vi "Analyse File to Prep DB.vi"(6 "Dummy Data 2":string, 7 "Dummy fill?":bool, 8 "error in (no error)":errorcluster, 9 "Dummy Data":string, 10 "Delimiter":string, 11 "Txt  file":path) -> (0 "error out":errorcluster, 1 "Value to be inserted":string, 2 "Table Elements":string, 3 "Table Schema":string)   [LabVIEW 2018]
panel:
  out "output array 2":string[][](array[string])
  in  "Quit":bool
  in  "User input Delimiter":string
  in  "Delimiter":enum16{"Tab", "Comma", "Space", "Ohters"}(ring)
  in  "Show":bool
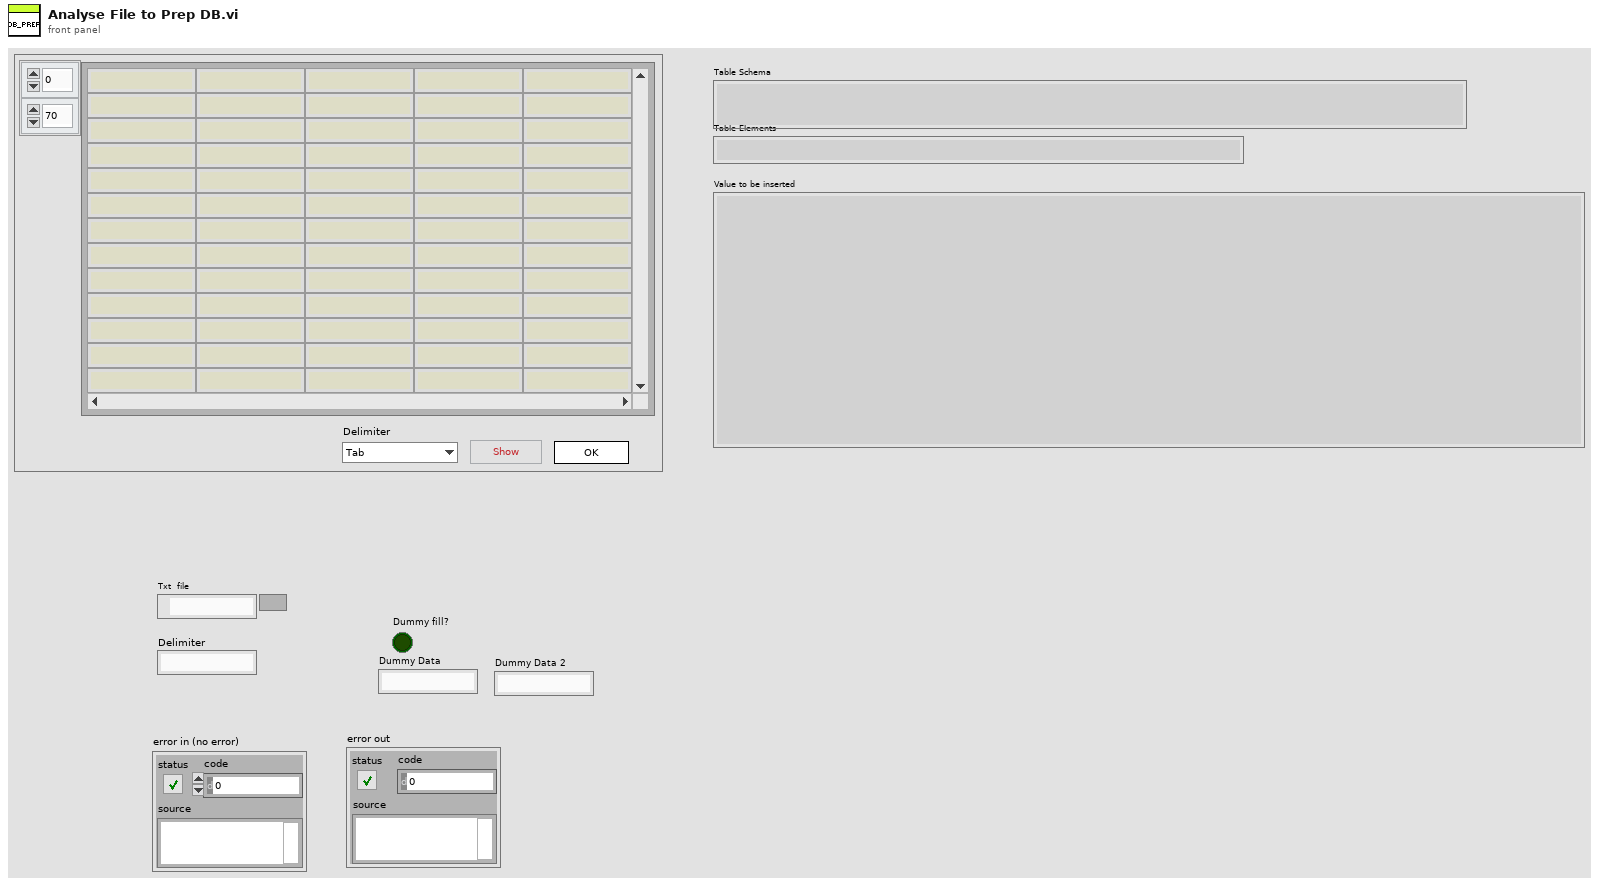
[diagram p1: front panel]
types:
  T1 = enum32{"Invalid", "Standard", "Closed", "Hidden", "Minimized", "Maximized"}
  T2 = enum32{"invalid app kind", "Development System", "Run Time System", "Student Edition", "Embedded LabVIEW", "Evaluation", "Custom"}
  T3 = cluster{"Core":cluster{"Current VI Reference":refnum<vi>, "Close Panel on Exit?":bool}, "Txt  file":path, "Delimiter":string, "Dummy fill?":bool}
  T4 = cluster{"Current VI Reference":refnum<vi>, "Close Panel on Exit?":bool}
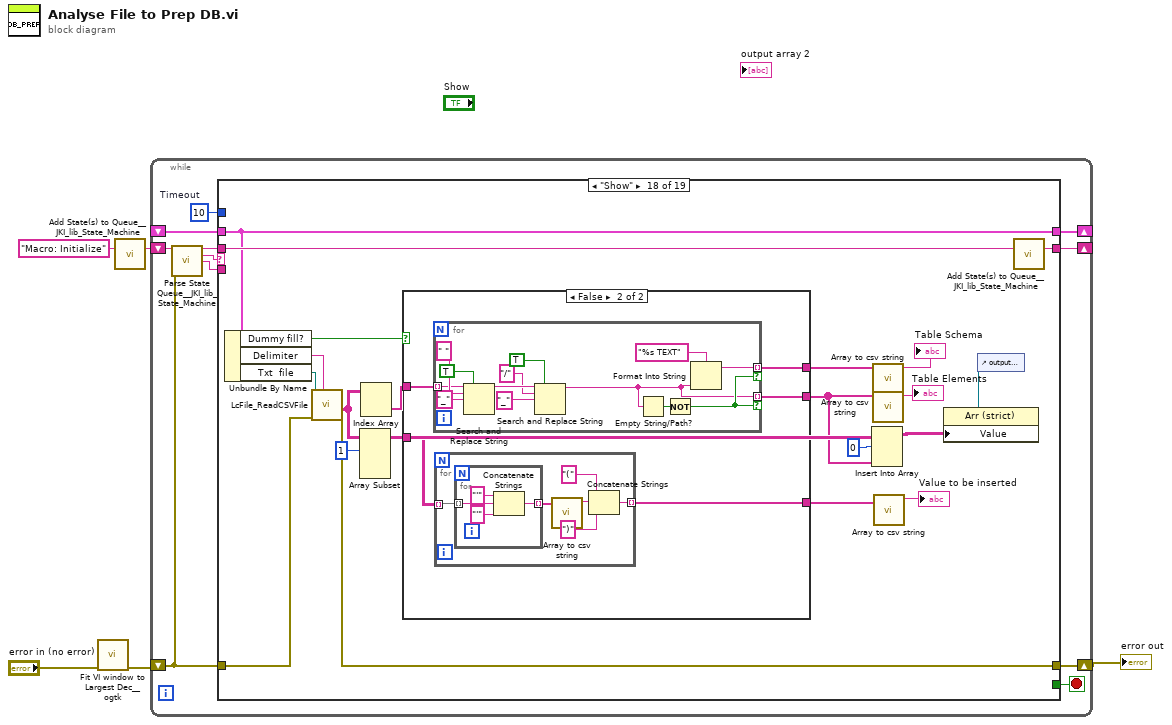
[diagram p0: block diagram]
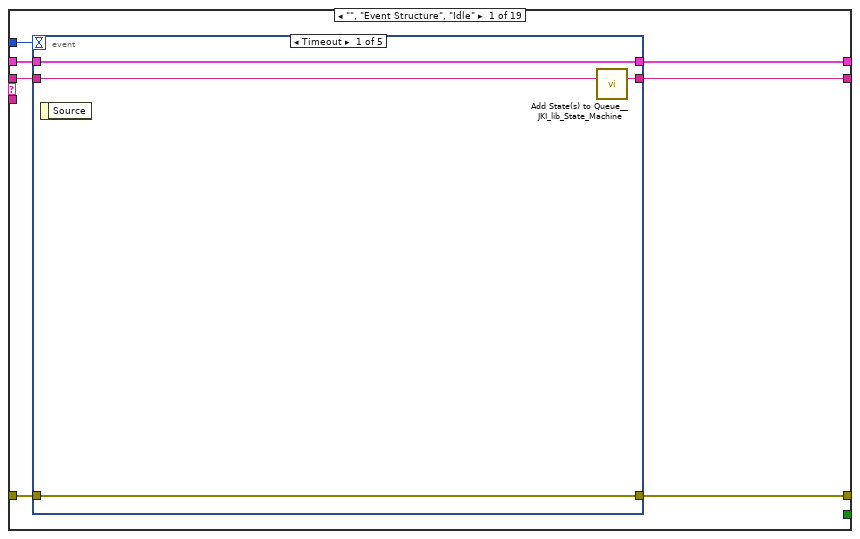
[diagram p2: hidden frame]
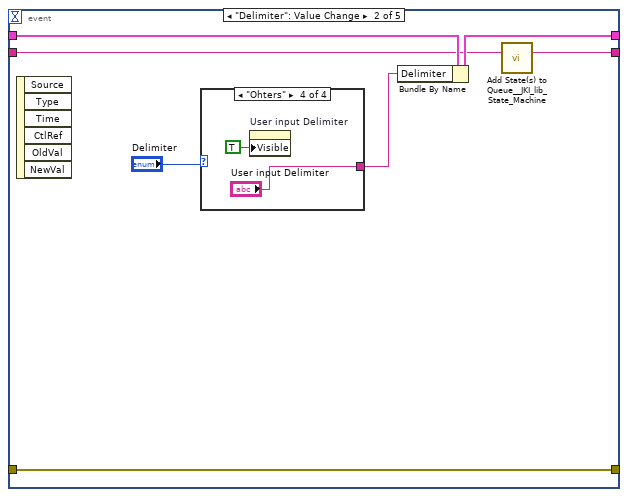
[diagram p3: hidden frame]
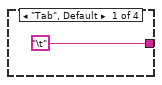
[diagram p4: hidden frame]
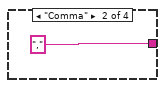
[diagram p5: hidden frame]
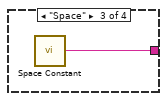
[diagram p6: hidden frame]
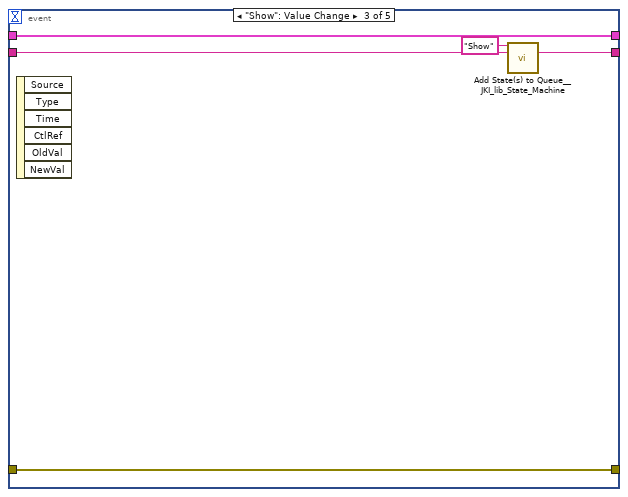
[diagram p7: hidden frame]
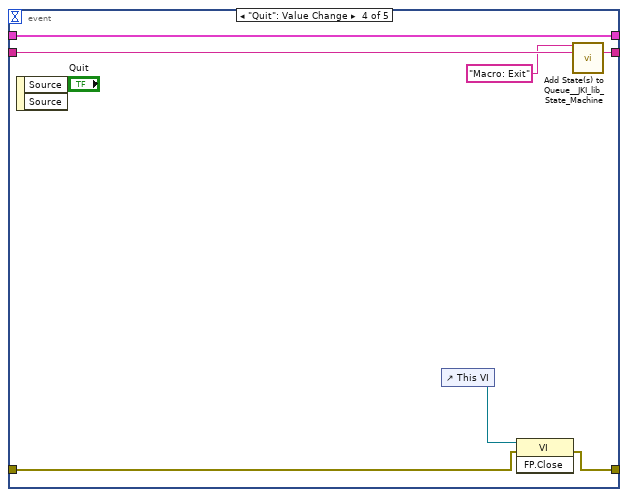
[diagram p8: hidden frame]
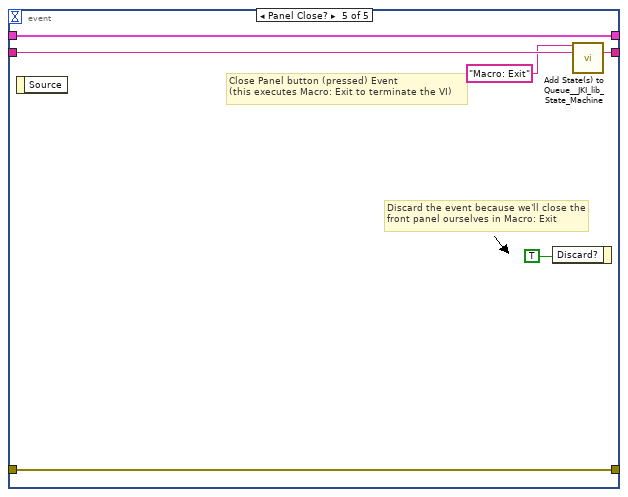
[diagram p9: hidden frame]
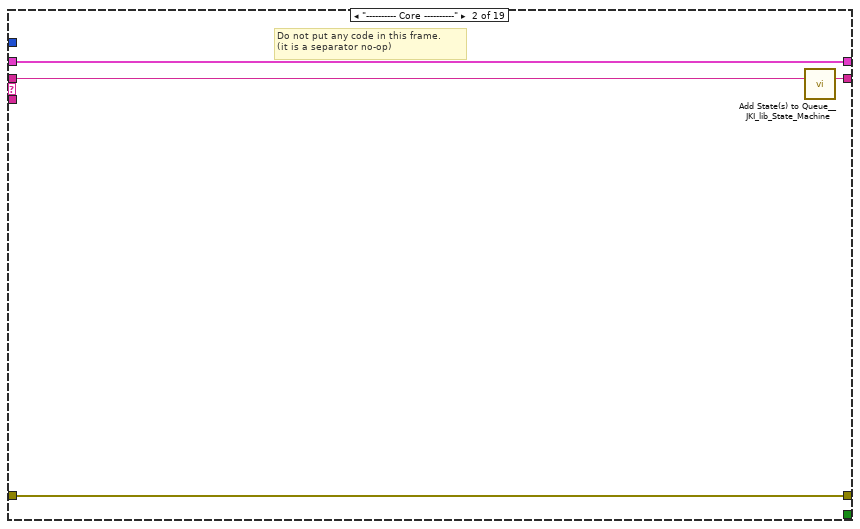
[diagram p10: hidden frame]
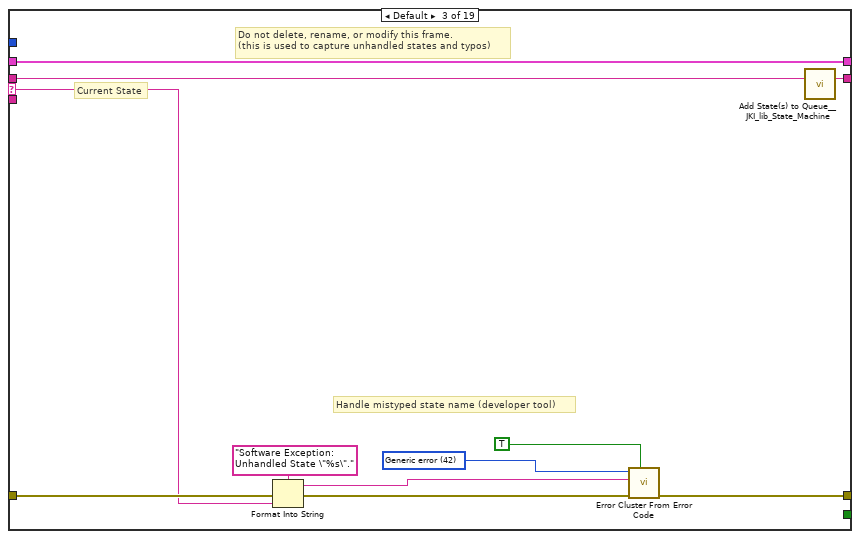
[diagram p11: hidden frame]
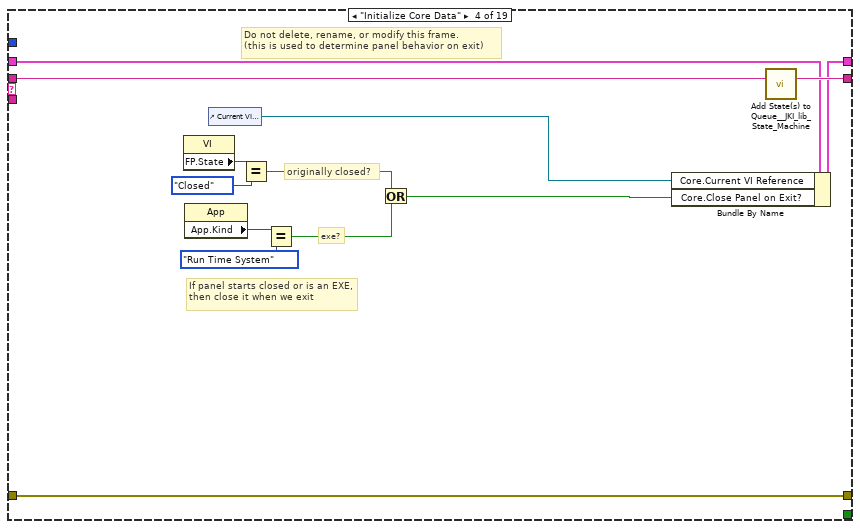
[diagram p12: hidden frame]
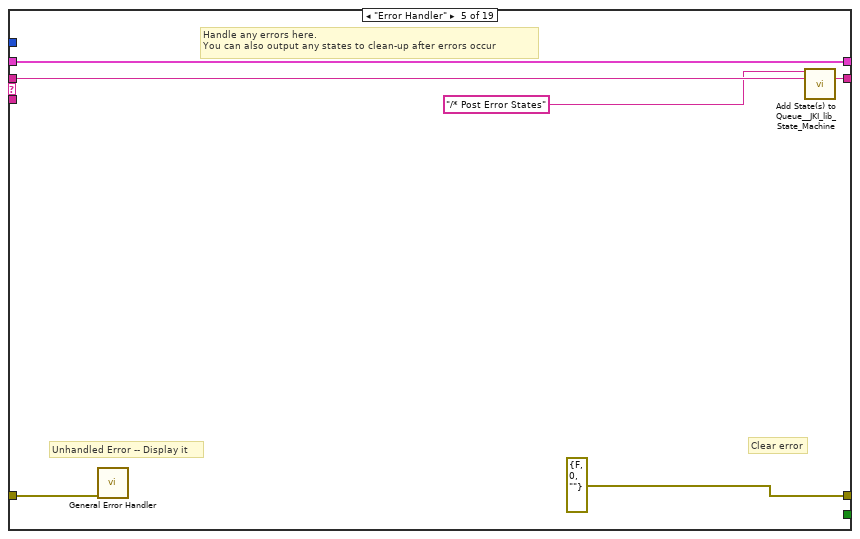
[diagram p13: hidden frame]
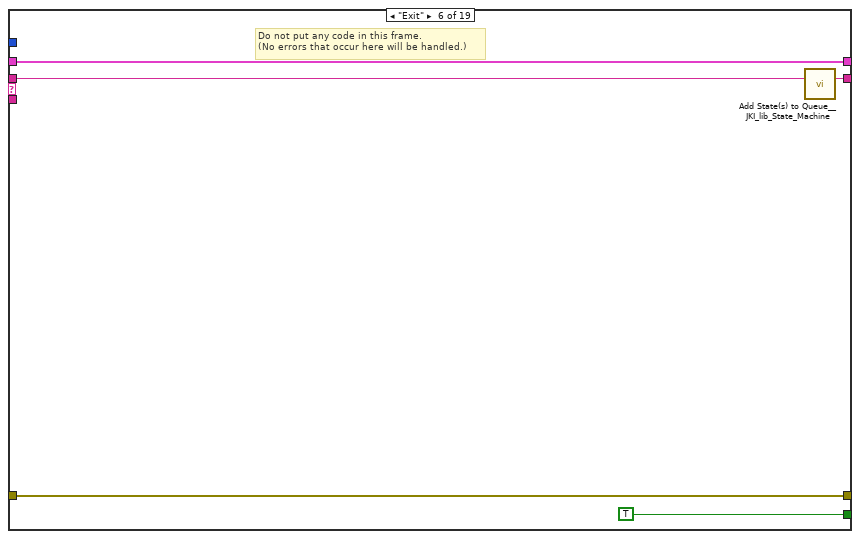
[diagram p14: hidden frame]
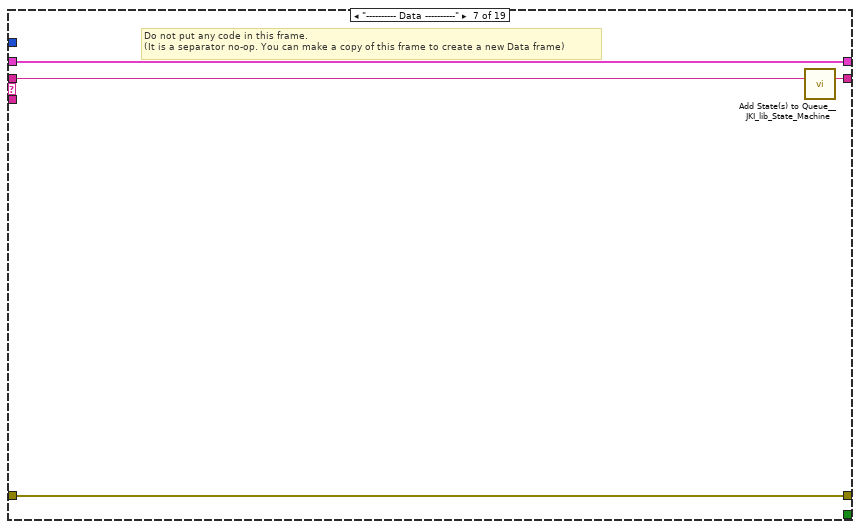
[diagram p15: hidden frame]
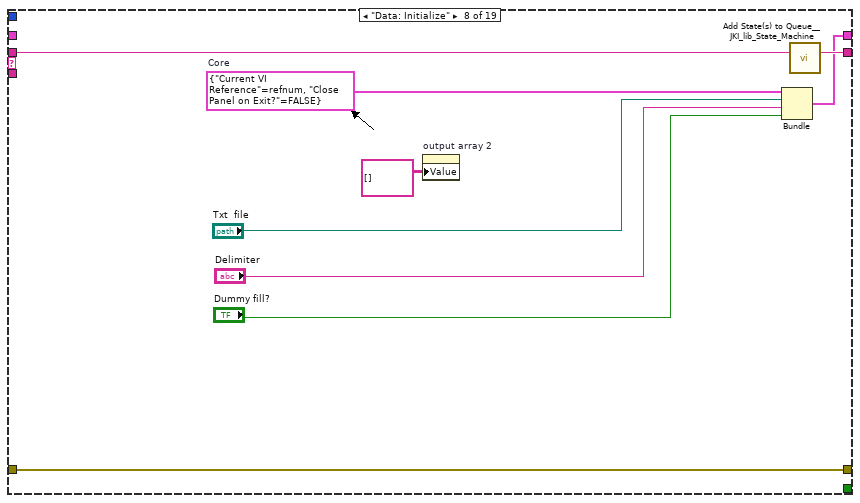
[diagram p16: hidden frame]
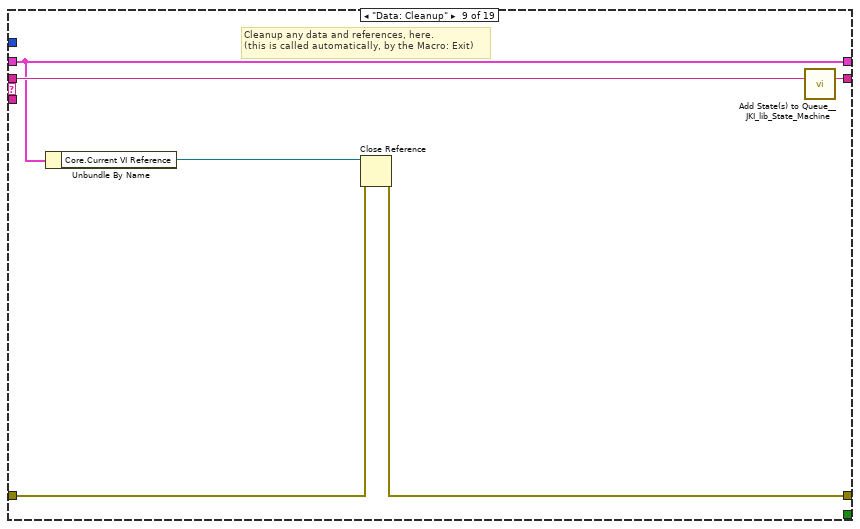
[diagram p17: hidden frame]
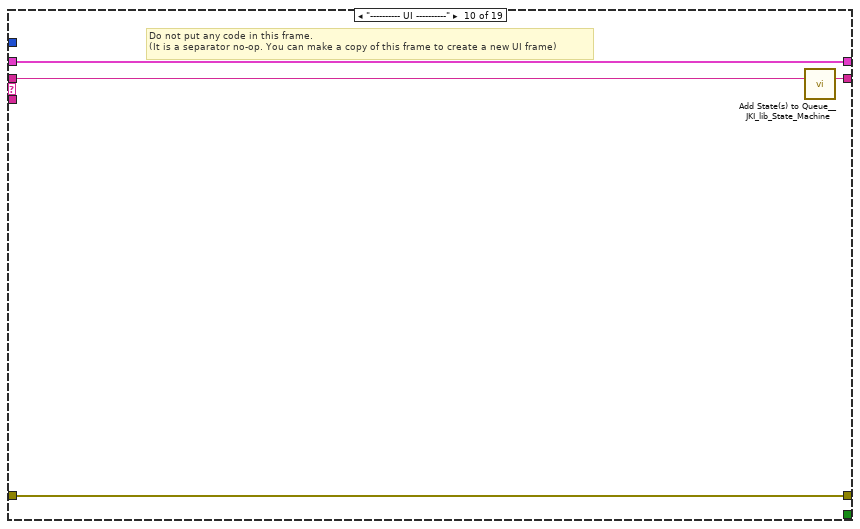
[diagram p18: hidden frame]
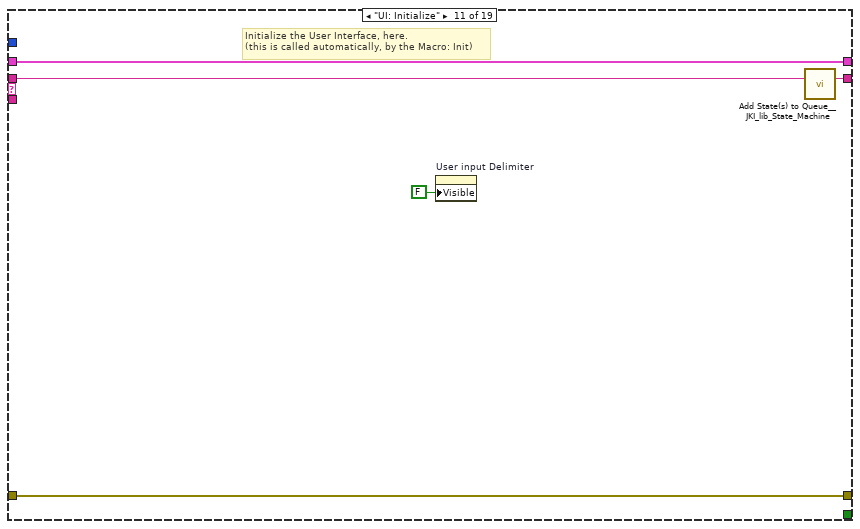
[diagram p19: hidden frame]
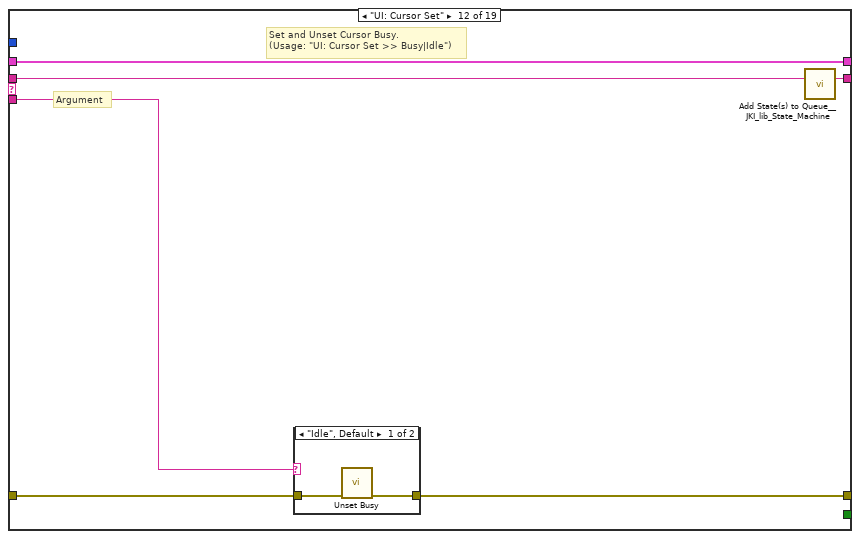
[diagram p20: hidden frame]
diagram:
  n1 = call <userlib>:"Fit VI window to Largest Dec__ogtk.vi"("error in (no error)"="error in (no error)") -> ("error out"=w3:errorcluster)  [unwired: 5 in, 1 out]
  n2 = call <vilib>:"Add State(s) to Queue__JKI_lib_State_Machine.vi"("State(s) in (\"\")"="Macro: Initialize") -> ("States Out"=w5:string)  [unwired: 14 in]
  n3 = while {
    shift-right: [w9] -> _
    shift-left: _ -> [w8]
    shift-right: [w12] -> w1
    shift-left: w3 -> [w6]
    shift-right: [w11] -> _
    shift-left: w5 -> [w13]
    stop <- w10 stop-if-true
    w7 = 10  # Timeout
    n4 = call <vilib>:"Parse State Queue__JKI_lib_State_Machine.vi"("State Queue"=w13, "Error In (no error)"=w6) -> ("Remaining States"=w15:string, "Current State"=w16:string, "Arguments"=w14:string)  [unwired: 11 in]
    n5 = case shown="\"Show\"" w16 {
      selector: w16 -> [_ _ w62 _ _ _ _ _ _ _ _ _ _ _ _ _ _ _ _]
      tunnel: w15 -> [w23 w61 w66 w85 w91 w96 w100 w109 w115 w119 w124 w130 w141 w210 w215 w225 w229 w250 w316]
      tunnel: w14 -> [_ _ _ _ _ _ _ _ _ _ _ w125 w135 _ _ _ _ _ _]
      tunnel: w8 -> [w21 w58 w64 w78 w88 w94 w97 _ w110 w116 w122 w128 w137 w207 w212 w222 w226 w237 w313]
      tunnel: [w20 w59 w68 w82 errorcluster {"status"=FALSE, "code"=0, "source"=""} ("error out") w93 w98 w106 w111 w117 w121 w126 w138 w208 w213 w223 w227 w230 w314] -> w12
      tunnel: w6 -> [w19 w59 w67 w82 w87 w93 w98 w106 w112 w117 w121 w127 w139 w208 w213 w223 w227 w232 w314]
      tunnel: [w22 w60 w65 w84 w90 w95 w99 w108 w114 w118 w123 w129 w140 w209 w214 w224 w228 w249 w315] -> w11
      tunnel: [_ _ _ _ _ TRUE _ _ _ _ _ _ _ _ _ _ _ _ _] -> w10
      tunnel: [w18 w58 w64 w83 w88 w94 w97 w107 w110 w116 w122 w128 w137 w207 w212 w222 w226 w237 w313] -> w9
      tunnel: w7 -> [w17 _ _ _ _ _ _ _ _ _ _ _ _ _ _ _ _ _ _]
      frame "", "Event Structure", "Idle" {
        n6 = event shown="[0] Timeout" {
          selector: _ -> [_ _ _ _ _]
          dyn-events: _ -> [_ _ _ _ _]
          timeout: w17 -> [_ _ _ _ _]
          tunnel: w23 -> [w27 w29 w42 w51 w57]
          tunnel: [w26 w30 w43 w50 w56] -> w22
          tunnel: w21 -> [w24 w33 w44 w49 w54]
          tunnel: [w25 w28 w41 w45 w55] -> w20
          tunnel: w19 -> [w25 w28 w41 w46 w55]
          tunnel: [w24 w31 w44 w49 w54] -> w18
          event Timeout {
            n7 = event-data() -> ()  [unwired: 1 in, 1 out]
            n8 = call <vilib>:"Add State(s) to Queue__JKI_lib_State_Machine.vi"("State(s) in (\"\")"=w27) -> ("States Out"=w26:string)  [unwired: 14 in]
          }
          event "Delimiter": Value Change {
            n9 = event-data() -> ()  [unwired: 1 in, 6 out]
            n10 = case shown="\"Ohters\"" "Delimiter" {
              tunnel: ["\t" "," w37 "User input Delimiter"] -> w32
              frame "Tab", Default {
              }
              frame "Comma" {
              }
              frame "Space" {
                n11 = call <vilib>:"Space Constant.vi"() -> ("String"=w37:string)
              }
              frame "Ohters" {
                n12 = property on="User input Delimiter" class="Str"("Visible"=TRUE) -> ()  [unwired: 2 in, 2 out]
              }
            }
            n13 = Bundle By Name(cluster=w33, "Delimiter"=w32) -> (w31:T3)
            n14 = call <vilib>:"Add State(s) to Queue__JKI_lib_State_Machine.vi"("State(s) in (\"\")"=w29) -> ("States Out"=w30:string)  [unwired: 14 in]
          }
          event "Show": Value Change {
            n15 = event-data() -> ()  [unwired: 1 in, 6 out]
            n16 = call <vilib>:"Add State(s) to Queue__JKI_lib_State_Machine.vi"("State(s) in Front (\"\")"="Show" ("State(s) in Front (\"\")"), "State(s) in (\"\")"=w42) -> ("States Out"=w43:string)  [unwired: 13 in]
          }
          event "Quit": Value Change {
            n17 = event-data() -> ()  [unwired: 1 in, 2 out]
            n18 = control-ref of="This VI"() -> (w47:refnum<vi>)
            n19 = invoke class="VI" method="FP.Close"(reference=w47, error in=w46) -> (error out=w45:errorcluster)  [unwired: 1 in, 2 out]
            n20 = call <vilib>:"Add State(s) to Queue__JKI_lib_State_Machine.vi"("State(s) in Front (\"\")"="Macro: Exit", "State(s) in (\"\")"=w51) -> ("States Out"=w50:string)  [unwired: 13 in]
          }
          event Panel Close? {
            # "Discard the event because we'll close the front panel ourselves in Macro: Exit"
            # "Close Panel button (pressed) Event\n(this executes Macro: Exit to terminate the VI)"
            n21 = event-data() -> ()  [unwired: 1 in, 1 out]
            n22 = event-data("Discard?"=TRUE) -> ()  [unwired: 1 in, 1 out]
            n23 = call <vilib>:"Add State(s) to Queue__JKI_lib_State_Machine.vi"("State(s) in Front (\"\")"="Macro: Exit", "State(s) in (\"\")"=w57) -> ("States Out"=w56:string)  [unwired: 13 in]
          }
        }
      }
      frame "---------- Core ----------" {
        # "Do not put any code in this frame.\n(it is a separator no-op)"
        n24 = call <vilib>:"Add State(s) to Queue__JKI_lib_State_Machine.vi"("State(s) in (\"\")"=w61) -> ("States Out"=w60:string)  [unwired: 14 in]
      }
      frame Default {
        w71 = 42 items=["No error", "Argument error", "Memory is full", "Out of zone", "End of file", "File already open", "Generic file I/O error", "File not found", "File permission error", "Disk is full", "Duplicate path", "Too many files open", "System feature not enabled", "Resource file not found", "Cannot add resource", "Resource not found", "Image not found", "Image memory error", "Pen does not exist", "Config type invalid", "Config token not found", "Config parse error", "Config memory error", "Bad external code format", "Bad external code offset", "External code not present", "Null window", "Destroy window error", "Null menu", "Print aborted", "Bad print record", "Print driver error", "Windows error during printing", "Memory error during printing", "Print dialog error", "Generic print error", "Invalid device refnum", "Device not found", "Device parameter error", "Device unit error", "Cannot open device", "Device call aborted", "Generic error", "Cancelled by user", "Object ID too low", "Object ID too high", "Object not in heap", "Unknown heap", "Unknown object (invalid DefProc)", "Unknown object (DefProc not in table)", "Message out of range", "Invalid (null) method", "Unknown message", "Manager call not supported", "Bad address", "Network operation in progress", "Network operation timed out", "Connection is busy", "Network attribute not supported", "Network error", "Address in use", "System out of memory", "Connection aborted", "Connection refused", "Not connected", "Already connected", "Connection closed", "Initialization error (interapplication manager)", "Bad occurrence", "Wait on unbound occurrence handler", "Occurrence queue overflow", "Datalog type conflict", "Unused", "Unrecognized type (interapplication manager)", "Memory corrupt", "Failed to make temporary DLL", "Old CIN version", "Drag socket not found", "Failed to load drop-object", "Failed to register OLE object", "Failed to release OLE object", "Format specifier type mismatch", "Unknown format specifier", "Too few format specifiers", "Too many format specifiers", "Scan failed", "Newer CIN version", "Error converting to variant", "Runtime menu error", "Password tampered", "Variant attribute not found", "Incompatible variant data type", "Event data is not available", "Event Store is not present", "Occurrence is not found", "Event Queue is not created", "Event info is not available", "Refnum passed is NULL", "Error retrieving Class GUID", "Error retrieving CoClass GUID", "Error retrieving TypeLib GUID.", "Bad built application magic bytes.", "Specific driver is different from the specific driver associated with the Logical Name.", "There is no session opened to the class driver.", "Max Error", "MAX - Error with config objects", "MAX - Error loading configuration", "MAX - Group not supported"]
        # "Current State"
        # "Do not delete, rename, or modify this frame.\n(this is used to capture unhandled states and typos)"
        # "Handle mistyped state name (developer tool)"
        n25 = Format Into String(format string="Software Exception: Unhandled State \"%s\"." ("message"), error in=w67, w62) -> (resulting string=w70:string, error out=w69:errorcluster)  [unwired: 1 in]
        n26 = call <vilib>:"Error Cluster From Error Code.vi"("show call chain? (False)"=TRUE, "error in (no error)"=w69, "error message (\"\")"=w70, "error code (0)"=w71) -> ("error out"=w68:errorcluster)  [unwired: 5 in]
        n27 = call <vilib>:"Add State(s) to Queue__JKI_lib_State_Machine.vi"("State(s) in (\"\")"=w66) -> ("States Out"=w65:string)  [unwired: 14 in]
      }
      frame "Initialize Core Data" {
        # "Do not delete, rename, or modify this frame.\n(this is used to determine panel behavior on exit)"
        # "originally closed?"
        # "exe?"
        # "If panel starts closed or is an EXE, then close it when we exit"
        n28 = property class="VI"() -> ("FP.State"=w75:T1)  [unwired: 2 in, 2 out]
        n29 = property class="App"() -> ("App.Kind"=w81:T2)  [unwired: 2 in, 2 out]
        n30 = control-ref of="Current VI Reference"() -> (w76:refnum<vi>)
        n31 = Equal?(x=w75, y=T1."Closed" ("Front Panel Window:State")) -> (x = y?=w73:bool)
        n32 = Equal?(x=w81, y=T2."Run Time System" ("Application:Kind")) -> (x = y?=w79:bool)
        n33 = Or(x=w73, y=w79) -> (x .or. y?=w77:bool)
        n34 = Bundle By Name(cluster=w78, "Core.Current VI Reference"=w76, "Core.Close Panel on Exit?"=w77) -> (w83:T3)
        n35 = call <vilib>:"Add State(s) to Queue__JKI_lib_State_Machine.vi"("State(s) in (\"\")"=w85) -> ("States Out"=w84:string)  [unwired: 14 in]
      }
      frame "Error Handler" {
        # "Unhandled Error -- Display it"
        # "Handle any errors here.\nYou can also output any states to clean-up after errors occur"
        # "Clear error"
        n36 = call <vilib>:"General Error Handler.vi"("error in (no error)"=w87) -> ()  [unwired: 10 in, 5 out]
        n37 = call <vilib>:"Add State(s) to Queue__JKI_lib_State_Machine.vi"("State(s) in Front (\"\")"="/* Post Error States", "State(s) in (\"\")"=w91) -> ("States Out"=w90:string)  [unwired: 13 in]
      }
      frame "Exit" {
        # "Do not put any code in this frame.\n(No errors that occur here will be handled.)"
        n38 = call <vilib>:"Add State(s) to Queue__JKI_lib_State_Machine.vi"("State(s) in (\"\")"=w96) -> ("States Out"=w95:string)  [unwired: 14 in]
      }
      frame "---------- Data ----------" {
        # "Do not put any code in this frame.\n(It is a separator no-op. You can make a copy of this frame to create a new Data frame)"
        n39 = call <vilib>:"Add State(s) to Queue__JKI_lib_State_Machine.vi"("State(s) in (\"\")"=w100) -> ("States Out"=w99:string)  [unwired: 14 in]
      }
      frame "Data: Initialize" {
        w105 = T4 {"Current VI Reference"=refnum, "Close Panel on Exit?"=FALSE}  # Core
        n40 = property on="output array 2" class="Arr (strict)"("Value"=string[][] [] ("output array 2")) -> ()  [unwired: 2 in, 2 out]
        n41 = Bundle("Core"=w105, "Txt  file"="Txt  file", "Delimiter"="Delimiter", "Dummy fill?"="Dummy fill?") -> (w107:T3)  [unwired: 1 in]
        n42 = call <vilib>:"Add State(s) to Queue__JKI_lib_State_Machine.vi"("State(s) in (\"\")"=w109) -> ("States Out"=w108:string)  [unwired: 14 in]
      }
      frame "Data: Cleanup" {
        # "Cleanup any data and references, here.\n(this is called automatically, by the Macro: Exit)"
        n43 = Unbundle By Name(w110) -> ("Core.Current VI Reference"=w113:refnum<vi>)
        n44 = Close Reference(reference=w113, error in (no error)=w112) -> (error out=w111:errorcluster)
        n45 = call <vilib>:"Add State(s) to Queue__JKI_lib_State_Machine.vi"("State(s) in (\"\")"=w115) -> ("States Out"=w114:string)  [unwired: 14 in]
      }
      frame "---------- UI ----------" {
        # "Do not put any code in this frame.\n(It is a separator no-op. You can make a copy of this frame to create a new UI frame)"
        n46 = call <vilib>:"Add State(s) to Queue__JKI_lib_State_Machine.vi"("State(s) in (\"\")"=w119) -> ("States Out"=w118:string)  [unwired: 14 in]
      }
      frame "UI: Initialize" {
        # "Initialize the User Interface, here.\n(this is called automatically, by the Macro: Init)"
        n47 = property on="User input Delimiter" class="Str"("Visible"=FALSE) -> ()  [unwired: 2 in, 2 out]
        n48 = call <vilib>:"Add State(s) to Queue__JKI_lib_State_Machine.vi"("State(s) in (\"\")"=w124) -> ("States Out"=w123:string)  [unwired: 14 in]
      }
      frame "UI: Cursor Set" {
        # "Argument"
        # "Set and Unset Cursor Busy.\n(Usage: \"UI: Cursor Set >> Busy|Idle\")"
        n49 = case shown="\"Idle\", Default" w125 {
          tunnel: w127 -> [w132 w134]
          tunnel: [w131 w133] -> w126
          frame "Idle", Default {
            n50 = call <vilib>:"Unset Busy.vi"("error in (no error)"=w132) -> ("error out"=w131:errorcluster)  [unwired: 10 in]
          }
          frame "Busy" {
            n51 = call <vilib>:"Set Busy.vi"("error in (no error)"=w134) -> ("error out"=w133:errorcluster)  [unwired: 9 in, 1 out]
          }
        }
        n52 = call <vilib>:"Add State(s) to Queue__JKI_lib_State_Machine.vi"("State(s) in (\"\")"=w130) -> ("States Out"=w129:string)  [unwired: 14 in]
      }
      frame "UI: Front Panel State" {
        # "Argument"
        # "Set Front Panel Open or Closed\n(Usage: \"UI: Front Panel State >> Open|Close\")"
        n53 = Unbundle By Name(w137) -> ("Core.Current VI Reference"=w136:refnum<vi>)
        n54 = case shown="\"Minimize\", \"Minimized\"" w135 {
          tunnel: w139 -> [w147 w162 w173 w186 w199]
          tunnel: [w149 w163 w175 w188 w201] -> w138
          tunnel: w136 -> [w148 w160 w174 w187 w200]
          frame "Open", "Standard", Default {
            w142 = T1."Standard" ("State")
            n55 = property class="VI"(reference=w148, error in=w147) -> (reference out=w145:refnum<vi>, error out=w146:errorcluster, "FP.State"=w144:T1)
            n56 = Not Equal?(x=w144, y=w142) -> (x != y?=w143:bool)
            n57 = case shown="True" w143 {
              tunnel: [w153 w155] -> w149
              tunnel: w146 -> [w152 w155]
              tunnel: w145 -> [w151 _]
              tunnel: w142 -> [w150 _]
              frame True {
                n58 = invoke class="VI" method="FP.Open"(reference=w151, error in=w152, "Activate"=TRUE, "State"=w150) -> (error out=w153:errorcluster)  [unwired: 1 in, 4 out]
              }
              frame False {
              }
            }
          }
          frame "Close", "Closed" {
            n59 = property class="VI"(reference=w160, error in=w162) -> (reference out=w159:refnum<vi>, error out=w161:errorcluster, "FP.State"=w157:T1)
            n60 = Not Equal?(x=w157, y=T1."Closed" ("Front Panel Window:State")) -> (x != y?=w156:bool)
            n61 = case shown="True" w156 {
              tunnel: [w164 w167] -> w163
              tunnel: w161 -> [w164 w166]
              tunnel: w159 -> [_ w165]
              frame False {
              }
              frame True {
                n62 = invoke class="VI" method="FP.Close"(reference=w165, error in=w166) -> (error out=w167:errorcluster)  [unwired: 1 in, 2 out]
              }
            }
          }
          frame "Hidden", "Hide" {
            w168 = T1."Hidden" ("State")
            n63 = property class="VI"(reference=w174, error in=w173) -> (reference out=w171:refnum<vi>, error out=w172:errorcluster, "FP.State"=w170:T1)
            n64 = Not Equal?(x=w170, y=w168) -> (x != y?=w169:bool)
            n65 = case shown="True" w169 {
              tunnel: [w179 w180] -> w175
              tunnel: w172 -> [w178 w180]
              tunnel: w171 -> [w177 _]
              tunnel: w168 -> [w176 _]
              frame True {
                n66 = invoke class="VI" method="FP.Open"(reference=w177, error in=w178, "State"=w176) -> (error out=w179:errorcluster)  [unwired: 2 in, 4 out]
              }
              frame False {
              }
            }
          }
          frame "Minimize", "Minimized" {
            w181 = T1."Minimized" ("State")
            n67 = property class="VI"(reference=w187, error in=w186) -> (reference out=w184:refnum<vi>, error out=w185:errorcluster, "FP.State"=w183:T1)
            n68 = Not Equal?(x=w183, y=w181) -> (x != y?=w182:bool)
            n69 = case shown="True" w182 {
              tunnel: [w192 w193] -> w188
              tunnel: w185 -> [w191 w193]
              tunnel: w184 -> [w190 _]
              tunnel: w181 -> [w189 _]
              frame True {
                n70 = invoke class="VI" method="FP.Open"(reference=w190, error in=w191, "State"=w189) -> (error out=w192:errorcluster)  [unwired: 2 in, 4 out]
              }
              frame False {
              }
            }
          }
          frame "Maximize", "Maximized" {
            w194 = T1."Maximized" ("State")
            n71 = property class="VI"(reference=w200, error in=w199) -> (reference out=w197:refnum<vi>, error out=w198:errorcluster, "FP.State"=w196:T1)
            n72 = Not Equal?(x=w196, y=w194) -> (x != y?=w195:bool)
            n73 = case shown="True" w195 {
              tunnel: [w205 w206] -> w201
              tunnel: w198 -> [w204 w206]
              tunnel: w197 -> [w203 _]
              tunnel: w194 -> [w202 _]
              frame True {
                n74 = invoke class="VI" method="FP.Open"(reference=w203, error in=w204, "State"=w202) -> (error out=w205:errorcluster)  [unwired: 2 in, 4 out]
              }
              frame False {
              }
            }
          }
        }
        n75 = call <vilib>:"Add State(s) to Queue__JKI_lib_State_Machine.vi"("State(s) in (\"\")"=w141) -> ("States Out"=w140:string)  [unwired: 14 in]
      }
      frame "---------- Macro ----------" {
        # "Do not put any code in this frame.\n(It is a separator no-op. You can make a copy of this frame to create a new Macro frame)"
        n76 = call <vilib>:"Add State(s) to Queue__JKI_lib_State_Machine.vi"("State(s) in (\"\")"=w210) -> ("States Out"=w209:string)  [unwired: 14 in]
      }
      frame "Macro: Initialize" {
        w211 = "Data: Initialize\nInitialize Core Data\nUI: Initialize\nUI: Front Panel State >> Open"  # Data: Initialize Initialize Core Data UI: Initialize UI: Front Panel State >> Open
        # "Initialization Macro\n(This is called once, when the VI starts)"
        n77 = call <vilib>:"Add State(s) to Queue__JKI_lib_State_Machine.vi"("State(s) in Front (\"\")"=w211, "State(s) in (\"\")"=w215) -> ("States Out"=w214:string)  [unwired: 13 in]
      }
      frame "Macro: Exit" {
        # "Exit Macro\n(This is called once, when the VI exits)"
        n78 = Unbundle By Name(w222) -> ("Core.Close Panel on Exit?"=w221:bool)
        n79 = Select(t="UI: Front Panel State >> Close", s=w221, f="") -> (s? t:f=w218:string)
        n80 = call <vilib>:"Add State(s) to Queue__JKI_lib_State_Machine.vi"("State(s) in (\"\")"=w218, "State(s) at Back (\"\")"="Data: Cleanup\nExit") -> ("States Out"=w216:string)  [unwired: 13 in]
        n81 = call <vilib>:"Add State(s) to Queue__JKI_lib_State_Machine.vi"("State(s) in Front (\"\")"=w216, "State(s) in (\"\")"=w225) -> ("States Out"=w224:string)  [unwired: 13 in]
      }
      frame "---------- New Category ----------" {
        # "Template Separator\n(You can make a copy of, or modify, this frame)"
        n82 = call <vilib>:"Add State(s) to Queue__JKI_lib_State_Machine.vi"("State(s) in (\"\")"=w229) -> ("States Out"=w228:string)  [unwired: 14 in]
      }
      frame "Show" {
        n83 = Unbundle By Name(w237) -> ("Dummy fill?"=w231:bool, "Delimiter"=w235:string, "Txt  file"=w236:path)
        n84 = call <userlib>:"LcFile_ReadCSVFile.vi"("delimiter (,)"=w235, "error in (no error)"=w232, "file path in"=w236) -> ("error out"=w230:errorcluster, "2-D array"=w242:string[][])  [unwired: 6 in, 1 out]
        n85 = Array Subset(array=w242, index (row)=1 ("index")) -> (w247:string[][])  [unwired: 3 in]
        n86 = Index Array(array=w242) -> (element=w243:string[])  [unwired: 2 in]
        n87 = case shown="False" w231 {
          tunnel: w247 -> [w261 w289]
          tunnel: [w254 w288] -> w246
          tunnel: [w260 w287] -> w245
          tunnel: w243 -> [w259 w286]
          tunnel: [w256 w285] -> w240
          frame True {
            n88 = for {
              tunnel: [w284] -> w258 mode=indexing if=w281
              tunnel: [w277] -> w255 mode=indexing if=w281
              tunnel: w259 -> [w278] mode=indexing
              n89 = Search and Replace String(input string=w278, search string=" ", replace string="_" ("replace string (\"\")")) -> (result string=w277:string)  [unwired: 5 in, 3 out]
              n90 = Empty String/Path?(string/path=w277) -> (empty?=w283:bool)
              n91 = Not(x=w283) -> (.not. x?=w281:bool)
              n92 = Format Into String(format string="%s TEXT", w277) -> (resulting string=w284:string)  [unwired: 2 in, 1 out]
            }
            n93 = for {
              tunnel: w261 -> [w266] mode=indexing
              tunnel: [w269] -> w260 mode=indexing
              tunnel: "Dummy Data" -> [w265]
              tunnel: "Dummy Data 2" -> [w262]
              n94 = Insert Into Array(array=w266, new element=w265) -> (w264:string[])  [unwired: 1 in]
              n95 = Insert Into Array(array=w264, new element=w262) -> (w263:string[])  [unwired: 1 in]
              n96 = for {
                tunnel: w263 -> [w274] mode=indexing
                tunnel: [w272] -> w268 mode=indexing
                n97 = Concatenate Strings("'" ("string"), w274, "'" ("string")) -> (w273:string)
                n98 = Concatenate Strings(w273) -> (w272:string)
              }
              n99 = call "Array to csv string.vi"("Array"=w268) -> ("spreadsheet string"=w267:string)  [unwired: 10 in]
              n100 = Concatenate Strings("(" ("string"), w267, ")" ("string")) -> (w269:string)
            }
            n101 = Insert Into Array(array=w258, new element="Date DATETIME,User TEXT" ("new element/subarray")) -> (w256:string[])  [unwired: 1 in]
            n102 = Insert Into Array(array=w255, new element="Date,User" ("new element/subarray")) -> (w254:string[])  [unwired: 1 in]
          }
          frame False {
            n103 = for {
              tunnel: [w312] -> w285 mode=indexing if=w309
              tunnel: [w304] -> w288 mode=indexing if=w309
              tunnel: w286 -> [w306] mode=indexing
              n104 = Search and Replace String(replace all?=TRUE ("replace all? (F)"), input string=w306, search string=" ", replace string="_" ("replace string (\"\")")) -> (result string=w301:string)  [unwired: 4 in, 3 out]
              n105 = Search and Replace String(replace all?=TRUE ("replace all? (F)"), input string=w301, search string="/", replace string="_" ("replace string (\"\")")) -> (result string=w304:string)  [unwired: 4 in, 3 out]
              n106 = Empty String/Path?(string/path=w304) -> (empty?=w311:bool)
              n107 = Not(x=w311) -> (.not. x?=w309:bool)
              n108 = Format Into String(format string="%s TEXT", w304) -> (resulting string=w312:string)  [unwired: 2 in, 1 out]
            }
            n109 = for {
              tunnel: w289 -> [w295] mode=indexing
              tunnel: [w292] -> w287 mode=indexing
              n110 = for {
                tunnel: w295 -> [w299] mode=indexing
                tunnel: [w296] -> w291 mode=indexing
                n111 = Concatenate Strings("'" ("string"), w299, "'" ("string")) -> (w296:string)
              }
              n112 = call "Array to csv string.vi"("Array"=w291) -> ("spreadsheet string"=w290:string)  [unwired: 10 in]
              n113 = Concatenate Strings("(" ("string"), w290, ")" ("string")) -> (w292:string)
            }
          }
        }
        n114 = Insert Into Array(array=w247, index (row)=0, new element=w246) -> (w233:string[][])  [unwired: 1 in]
        n115 = call "Array to csv string.vi"("Array"=w240) -> ("spreadsheet string"=→"Table Schema":string)  [unwired: 10 in]
        n116 = call "Array to csv string.vi"("Array"=w246) -> ("spreadsheet string"=→"Table Elements":string)  [unwired: 10 in]
        n117 = call "Array to csv string.vi"("Array"=w245) -> ("spreadsheet string"=→"Value to be inserted":string)  [unwired: 10 in]
        n118 = control-ref of="output array 2"() -> (w234:refnum<vi>)
        n119 = property class="Arr (strict)"(reference=w234, "Value"=w233) -> ()  [unwired: 1 in, 2 out]
        n120 = call <vilib>:"Add State(s) to Queue__JKI_lib_State_Machine.vi"("State(s) in (\"\")"=w250) -> ("States Out"=w249:string)  [unwired: 14 in]
      }
      frame "New Category: 2" {
        # "Your code here.\n(You can make a copy of, or modify, this frame)"
        n121 = call <vilib>:"Add State(s) to Queue__JKI_lib_State_Machine.vi"("State(s) in (\"\")"=w316) -> ("States Out"=w315:string)  [unwired: 14 in]
      }
    }
  }
  "error out" <- w1
